vi "fpga_LineInputs-TBank5-1dead.vi"() -> (0 "DataLines":T1)   [LabVIEW 2011]
uses:
  <vilib>/rvi/eio/common/nirviEmuTemplateMethod_errors.vi
  <vilib>/eio/EIONode/EIONode.xnode
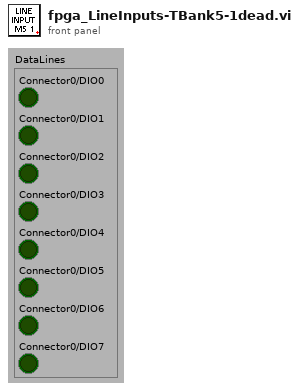
[diagram p1: front panel]
types:
  T1 = cluster{"Connector0/DIO0":bool, "Connector0/DIO1":bool, "Connector0/DIO2":bool, "Connector0/DIO3":bool, "Connector0/DIO4":bool, "Connector0/DIO5":bool, "Connector0/DIO6":bool, "Connector0/DIO7":bool}
  T2 = cluster{bool, bool, "Connector2/DIO29":bool, "Connector1/DIO39":bool, "Connector2/DIO9":bool, "Connector1/DIO13":bool, "Connector2/DIO12":bool, "Connector1/DIO14":bool}
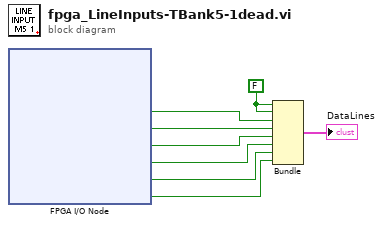
[diagram p0: block diagram]
diagram:
  w2 = FALSE
  n1 = xnode "FPGA I/O Node"() -> ("Connector2/DIO29"=w8:bool, "Connector1/DIO39"=w7:bool, "Connector2/DIO9"=w6:bool, "Connector1/DIO13"=w5:bool, "Connector2/DIO12"=w4:bool, "Connector1/DIO14"=w3:bool)  [unwired: 8 in, 10 out]
  n2 = Bundle(w2, w2, "Connector2/DIO29"=w8, "Connector1/DIO39"=w7, "Connector2/DIO9"=w6, "Connector1/DIO13"=w5, "Connector2/DIO12"=w4, "Connector1/DIO14"=w3) -> (→"DataLines":T2)  [unwired: 1 in]
